vi "ExFileReadNConvertToU16.vi"() -> ()   [LabVIEW 2010]
panel:
  in  "Full File Name":path=path "C:/Program Files/SIToolKit/LabVIEW/Data Files/Color.SPE"
  in  "?":bool
  in  "FileType":u32=67371008
  out "error out":errorcluster
  in  "error in (no error)":errorcluster
  # "ExReadFileNconvertToU16.vi\nThis example will read in a file of the\nselected data type and display as u16 frame.\nWhen finished viewing data, make sure to\nuse the STOP button to close the display."
  # "File Types:\nSPE = 67371008\nTIF   = 67174400\nPMI  = 67436544"
  # "Browse match pattern is set to *.spe.  Modify this if different file type is needed."
  # "This will properly close\nthe image and\ndeallocate memory."
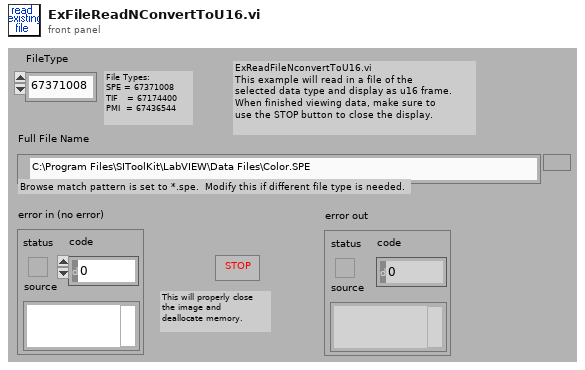
[diagram p1: front panel]
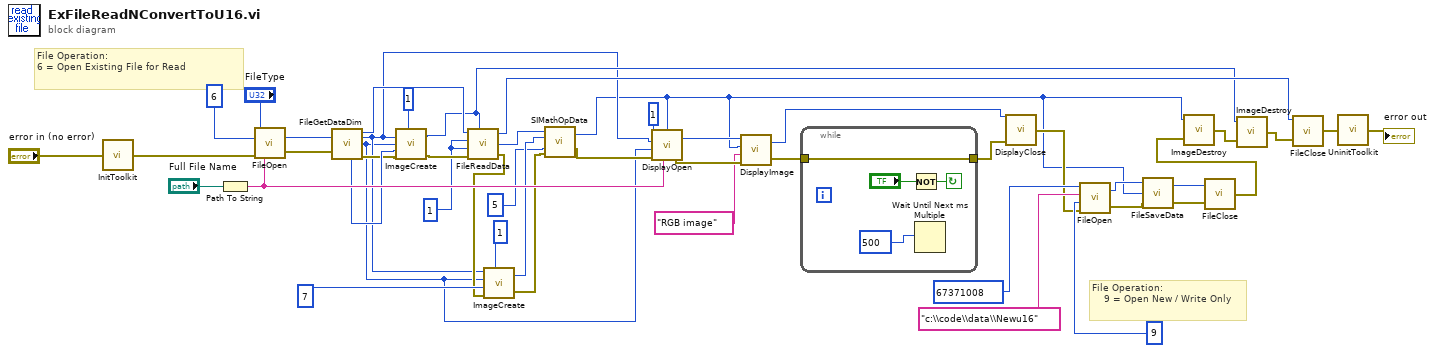
[diagram p0: block diagram]
diagram:
  w33 = 1
  # "File Operation:\n    9 = Open New / Write Only"
  # "File Operation:\n6 = Open Existing File for Read"
  n1 = call <userlib>:"InitToolkit.vi"("error in"="error in (no error)") -> ("error out"=w45:errorcluster)
  n2 = Path To String(path="Full File Name") -> (string=w36:string)
  n3 = call <userlib>:"FileOpen.vi"("error in"=w45, "File Operations"=u32 6 ("File Operation"), "FileName"=w36, "File Type"="FileType") -> ("error out"=w43:errorcluster, "File Handle"=w42:u32)
  n4 = call <userlib>:"FileGetDataDim.vi"("File Handle"=w42, "error in"=w43) -> ("Data Type"=w23:u32, "File Handle"=w35:u32, "X dim"=w3:u32, "Y dim"=w2:u32, "error out"=w19:errorcluster)  [unwired: 1 out]
  n5 = call <userlib>:"ImageCreate.vi"("X dimension"=w3, "Y dimension"=w2, "Data Type"=w23, "error in"=w19, "Number Of Frames"=1) -> ("Image Handle"=w25:u32, "error out"=w34:errorcluster)
  n6 = call <userlib>:"FileReadData.vi"("File Handle"=w35, "Start Frame"=w33, "End Frame"=w33, "error in"=w34, "Image Handle"=w25) -> ("File Handle"=w32:u32, "Image Handle"=w16:u32, "error out"=w20:errorcluster)
  n7 = call <userlib>:"ImageCreate.vi"("X dimension"=w3, "Y dimension"=w2, "Data Type"=7, "error in"=w20, "Number Of Frames"=1) -> ("Image Handle"=w17:u32, "error out"=w18:errorcluster)
  n8 = call <userlib>:"SIMathOpData.vi"("error in (no error)"=w18, "Operation"=5, "Result Handle"=w17, "Data Handle"=w16) -> ("error out"=w14:errorcluster, "Result Handle"=w1:u32)
  n9 = call <userlib>:"DisplayOpen.vi"("Display Title"=w36, "Image Handle"=w1, "error in"=w14, "Display Height"=w2, "Display Width"=w3, "Display Type"=1) -> ("error out"=w31:errorcluster, "Display Handle"=w30:u32)
  n10 = call <userlib>:"DisplayImage.vi"("error in"=w31, "Title"="RGB image", "Image Handle"=w1, "Display Handle"=w30) -> ("error out"=w24:errorcluster, "Display Handle"=w29:u32)
  n11 = while {
    tunnel: w24 -> [w48]
    tunnel: [w48] -> w6
    stop <- w50 continue-if-true
    n12 = Not(x="?") -> (.not. x?=w50:bool)
    n13 = Wait Until Next ms Multiple(millisecond multiple=500) -> ()  [unwired: 1 out]
  }
  n14 = call <userlib>:"DisplayClose.vi"("error in"=w6, "Display Handle"=w29) -> ("error out"=w5:errorcluster)
  n15 = call <userlib>:"FileOpen.vi"("error in"=w5, "File Operations"=9, "FileName"="c:\\code\\data\\Newu16", "File Type"=67371008) -> ("error out"=w13:errorcluster, "File Handle"=w11:u32)
  n16 = call <userlib>:"FileSaveData.vi"("error in"=w13, "Image Handle"=w1, "File Handle"=w11) -> ("error out"=w12:errorcluster, "File Handle"=w10:u32)
  n17 = call <userlib>:"FileClose.vi"("error in"=w12, "File Handle"=w10) -> ("error out"=w4:errorcluster)
  n18 = call <userlib>:"ImageDestroy.vi"("error in"=w4, "Data handle"=w1) -> ("error out"=w28:errorcluster)
  n19 = call <userlib>:"ImageDestroy.vi"("error in"=w28, "Data handle"=w25) -> ("error out"=w27:errorcluster)
  n20 = call <userlib>:"FileClose.vi"("error in"=w27, "File Handle"=w32) -> ("error out"=w39:errorcluster)
  n21 = call <userlib>:"UninitToolkit.vi"("error in"=w39) -> ("error out"=→"error out":errorcluster)
